vi "List VIs without Test Coverage.vi"(8 "error in (no error)":errorcluster, 9 "Tests Root":path, 10 "Source Root":path) -> (0 "error out":errorcluster, 1 "Test VIs":path[](array[path]), 2 "VIs without test coverage":string[](array[string]))   [LabVIEW 2020]
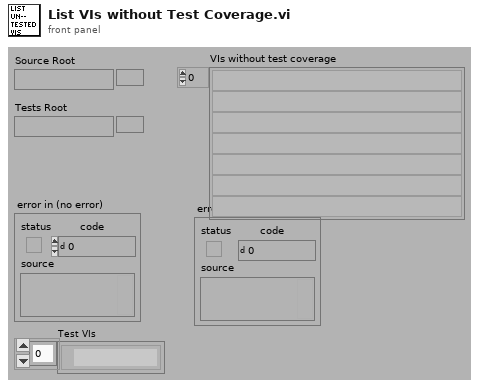
[diagram p1: front panel]
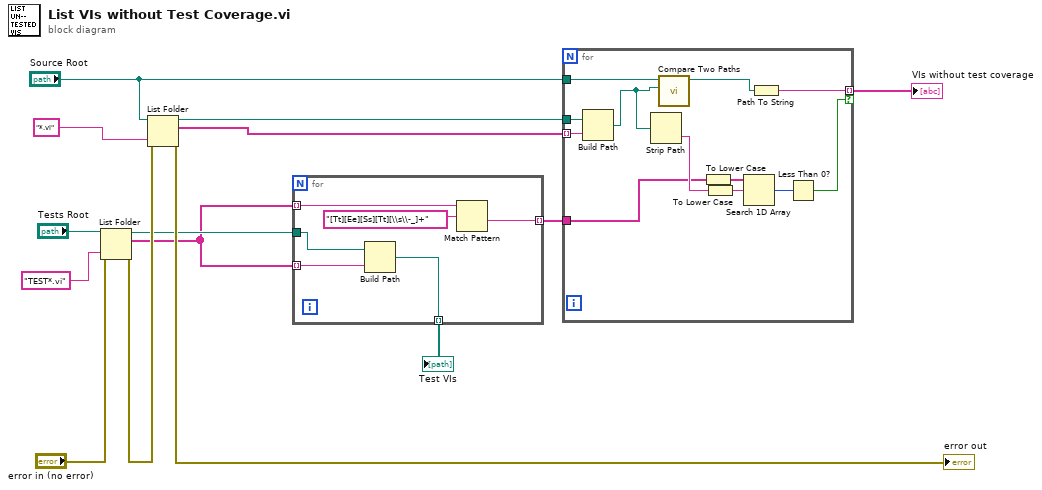
[diagram p0: block diagram]
diagram:
  n1 = List Folder(path="Tests Root", pattern="TEST*.vi", error in="error in (no error)") -> (path out=w3:path, filenames=w2:string[], error out=w10:errorcluster)  [unwired: 1 in, 1 out]
  n2 = List Folder(path="Source Root", pattern="*.vi", error in=w10) -> (path out=w5:path, filenames=w4:string[], error out=→"error out":errorcluster)  [unwired: 1 in, 1 out]
  n3 = for {
    tunnel: w2 -> [w20] mode=indexing
    tunnel: [w18] -> w9 mode=indexing
    tunnel: w3 -> [w17]
    tunnel: w2 -> [w16] mode=indexing
    tunnel: [w15] -> w1 mode=indexing
    n4 = Build Path(base path=w17, name or relative path=w16) -> (appended path=w15:path)
    n5 = Match Pattern(string=w20, regular expression="[Tt][Ee][Ss][Tt][\\s\\-_]+") -> (after substring=w18:string)  [unwired: 1 in, 3 out]
  }
  "Test VIs" <- w1
  n6 = for {
    tunnel: w9 -> [w31]
    tunnel: "Source Root" -> [w24]
    tunnel: [w29] -> w14 mode=indexing if=w26
    tunnel: w5 -> [w28]
    tunnel: w4 -> [w27] mode=indexing
    n7 = Build Path(base path=w28, name or relative path=w27) -> (appended path=w23:path)
    n8 = Strip Path(path=w23) -> (name=w32:string)  [unwired: 1 out]
    n9 = call <vilib>:"Compare Two Paths.vi"("Path 2"=w23, "Path 1"=w24) -> ("Relative Path from 1 to 2"=w25:path)  [unwired: 6 in, 3 out]
    n10 = To Lower Case(string=w31) -> (all lower case string=w21:string[])
    n11 = To Lower Case(string=w32) -> (all lower case string=w22:string)
    n12 = Search 1D Array(1D array=w21, element=w22) -> (index of element=w30:i32)  [unwired: 1 in]
    n13 = Path To String(path=w25) -> (string=w29:string)
    n14 = Less Than 0?(x=w30) -> (x < 0?=w26:bool)
  }
  "VIs without test coverage" <- w14
